vi "Export Custom Device Configuration.vi"(6 "operation":T1(ring)=enum."replace or create with confirmation", 7 "Root? (T)":bool=TRUE, 8 "error in (no error)":errorcluster, 9 "File Interface in":refnum<class "File Interface.lvclass">, 10 "Path":path, 11 "ID":u64) -> (0 "error out":errorcluster, 3 "ID out":u64)   [LabVIEW 2020, in "ImportExport.lvlib"]
doc: "ExportCDConfig.vi saves a configuration file (.dat) that can be later loaded using ImportCDConfig.vi. This configuration file includes the values for the properties of each Section, Channel, or Waveform in your Custom Device. You can add this functionality as a Button, Runtime Menu, or as a property for one of your Channels."
uses:
  ImportExport.lvlib
  File Interface Class/File Interface.lvclass
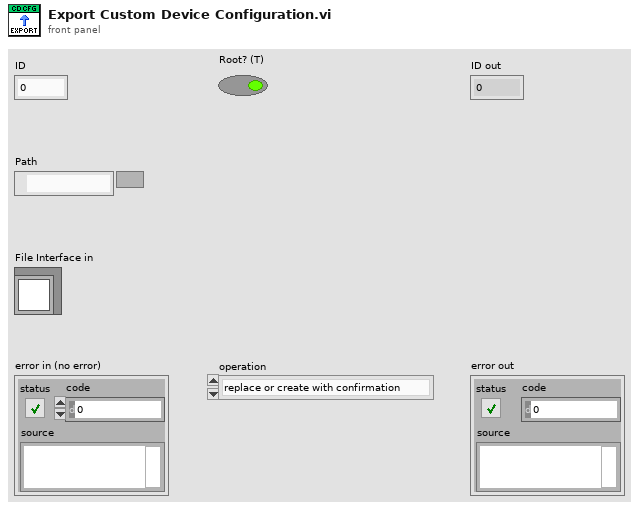
[diagram p1: front panel]
types:
  T1 = enum16{"open", "replace", "create", "open or create", "replace or create", "replace or create with confirmation"}
  T2 = typedef "Advanced System Definition.lvlib/SysDef.Export.ctl" = cluster{"Version":string, "Tree":T3[]}
  T3 = typedef "Advanced System Definition.lvlib/TreeItem.ctl" = cluster{"Item Info":T4, "Parent Path":string[], "Properties":T9[]}
  T4 = typedef "Advanced System Definition.lvlib/TreeItem.Info.ctl" = cluster{"Name":string, "Description":string, "GUID":string, "Is Channel":bool, "Channel":T5, "Is Waveform":bool, "Waveform":T7}
  T5 = typedef "Custom Device API.lvlib/Custom Device Channel.ctl" = cluster{"Type":T6, "Units":string, "Default Value":dbl, "Faultable":bool, "Scalable":bool}
  T6 = typedef "Custom Device API.lvlib/Custom Device Channel Type.ctl" = enum16{"Input", "Output"}
  T7 = typedef "Custom Device API.lvlib/Custom Device Waveform.ctl" = cluster{"Data Type":T8, "Units":string}
  T8 = typedef "Custom Device API.lvlib/Custom Device Waveform DataType.ctl" = enum16{"Double", "Complex Double"}
  T9 = typedef "Advanced System Definition.lvlib/TreeItem.Property.ctl" = cluster{"Name":string, "Type":i32, "Value":variant}
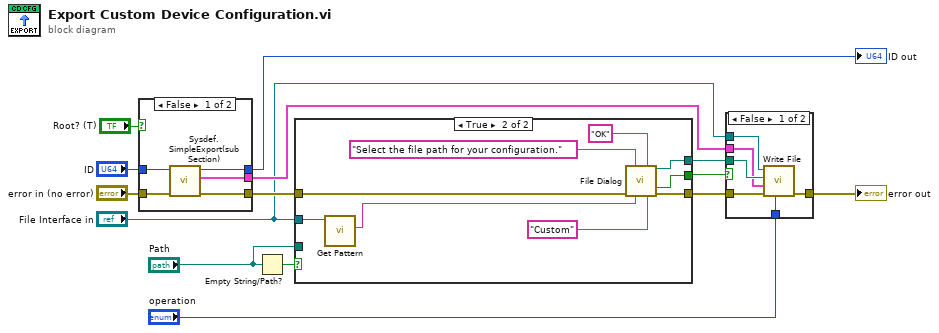
[diagram p0: block diagram]
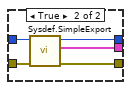
[diagram p2: hidden frame]
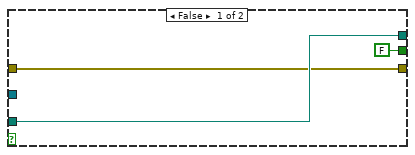
[diagram p3: hidden frame]
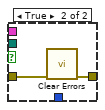
[diagram p4: hidden frame]
diagram:
  n1 = case shown="False" "Root? (T)" {
    tunnel: [w16 w24] -> w14
    tunnel: [w15 w20] -> w13
    tunnel: "error in (no error)" -> [w18 w23]
    tunnel: "ID" -> [w19 w22]
    tunnel: [w17 w21] -> w10
    frame False {
      n2 = call "Sysdef.SimpleExport(subSection).vi"("error in (no error)"=w18, "ID"=w19) -> ("error out"=w16:errorcluster, "Exported Section"=w15:T2, "ID out"=w17:u64)  [unwired: 7 in]
    }
    frame True {
      n3 = call "Sysdef.SimpleExport.vi"("error in (no error)"=w23, "ID"=w22) -> ("error out"=w24:errorcluster, "Export"=w20:T2, "ID out"=w21:u64)  [unwired: 7 in]
    }
  }
  "ID out" <- w10
  n4 = Empty String/Path?(string/path="Path") -> (empty?=w5:bool)
  n5 = case shown="True" w5 {
    tunnel: w14 -> [w26 w36]
    tunnel: "File Interface in" -> [_ w35]
    tunnel: [FALSE ("cancelled") w31] -> w8
    tunnel: [w26 w30] -> w7
    tunnel: [w27 w29] -> w6
    tunnel: "Path" -> [w27 _]
    frame False {
    }
    frame True {
      n6 = call-dynamic "Get Pattern.vi"("File Interface in"=w35) -> ("file extension"=w28:string)  [unwired: 10 in]
      n7 = call "File Dialog"("prompt"="Select the file path for your configuration.", "button label"="OK", "error in"=w36, "pattern (all files)"=w28, "pattern label"="Custom") -> ("selected path"=w29:path, "cancelled"=w31:bool, "error out"=w30:errorcluster)  [unwired: 7 in, 1 out]
    }
  }
  n8 = case shown="False" w8 {
    tunnel: [w38 w43] -> w9
    tunnel: w7 -> [w39 w44]
    tunnel: w6 -> [w41 _]
    tunnel: w13 -> [w40 _]
    tunnel: "File Interface in" -> [w42 _]
    tunnel: "operation" -> [w37 _]
    frame False {
      n9 = call-dynamic "Write File.vi"("operation"=w37, "error in (no error)"=w39, "Data"=w40, "datalog path (use dialog)"=w41, "File Interface in"=w42) -> ("error out"=w38:errorcluster)  [unwired: 6 in]
    }
    frame True {
      n10 = call <vilib>:"Clear Errors.vi"("error in (no error)"=w44) -> ("error out"=w43:errorcluster)  [unwired: 5 in, 1 out]
    }
  }
  "error out" <- w9
